vi "Runrate2.vi"() -> ()   [LabVIEW 2012]
uses:
  <vilib>/addons/database/Auxilliary.llb/DB Tools Cursor Type.ctl
  <vilib>/Utility/NIReport.llb/NI_report.lvclass
  <vilib>/addons/database/Connection.llb/DB Tools Open Connec (Path).vi
  <vilib>/addons/database/Connection.llb/Conn Execute.vi
  <vilib>/addons/database/Recordset.llb/Rec Fetch Recordset Data (R).vi
  <vilib>/addons/database/Recordset.llb/Rec Destroy - Connection.vi
  <vilib>/Utility/NIReport.llb/Append Text Table to Report (wrap).vi
  <vilib>/addons/database/_DB Variant To Data/Database Variant To Data.xnode
  <vilib>/addons/database/NI_Database_API.lvlib
  <vilib>/Utility/NIReport.llb/Excel/NI_Excel.lvclass
  <vilib>/addons/_office/NI_ReportGenerationToolkit.lvlib
panel:
  out "error out 2":errorcluster
  in  "Table Control":string[][](table)
  out "error out":errorcluster
  out "recordset data":variant[][](array[variant])
  out "array":string[][](array[string])
  out "transposed array":string[][](array[string])
  out "concatenated string":string
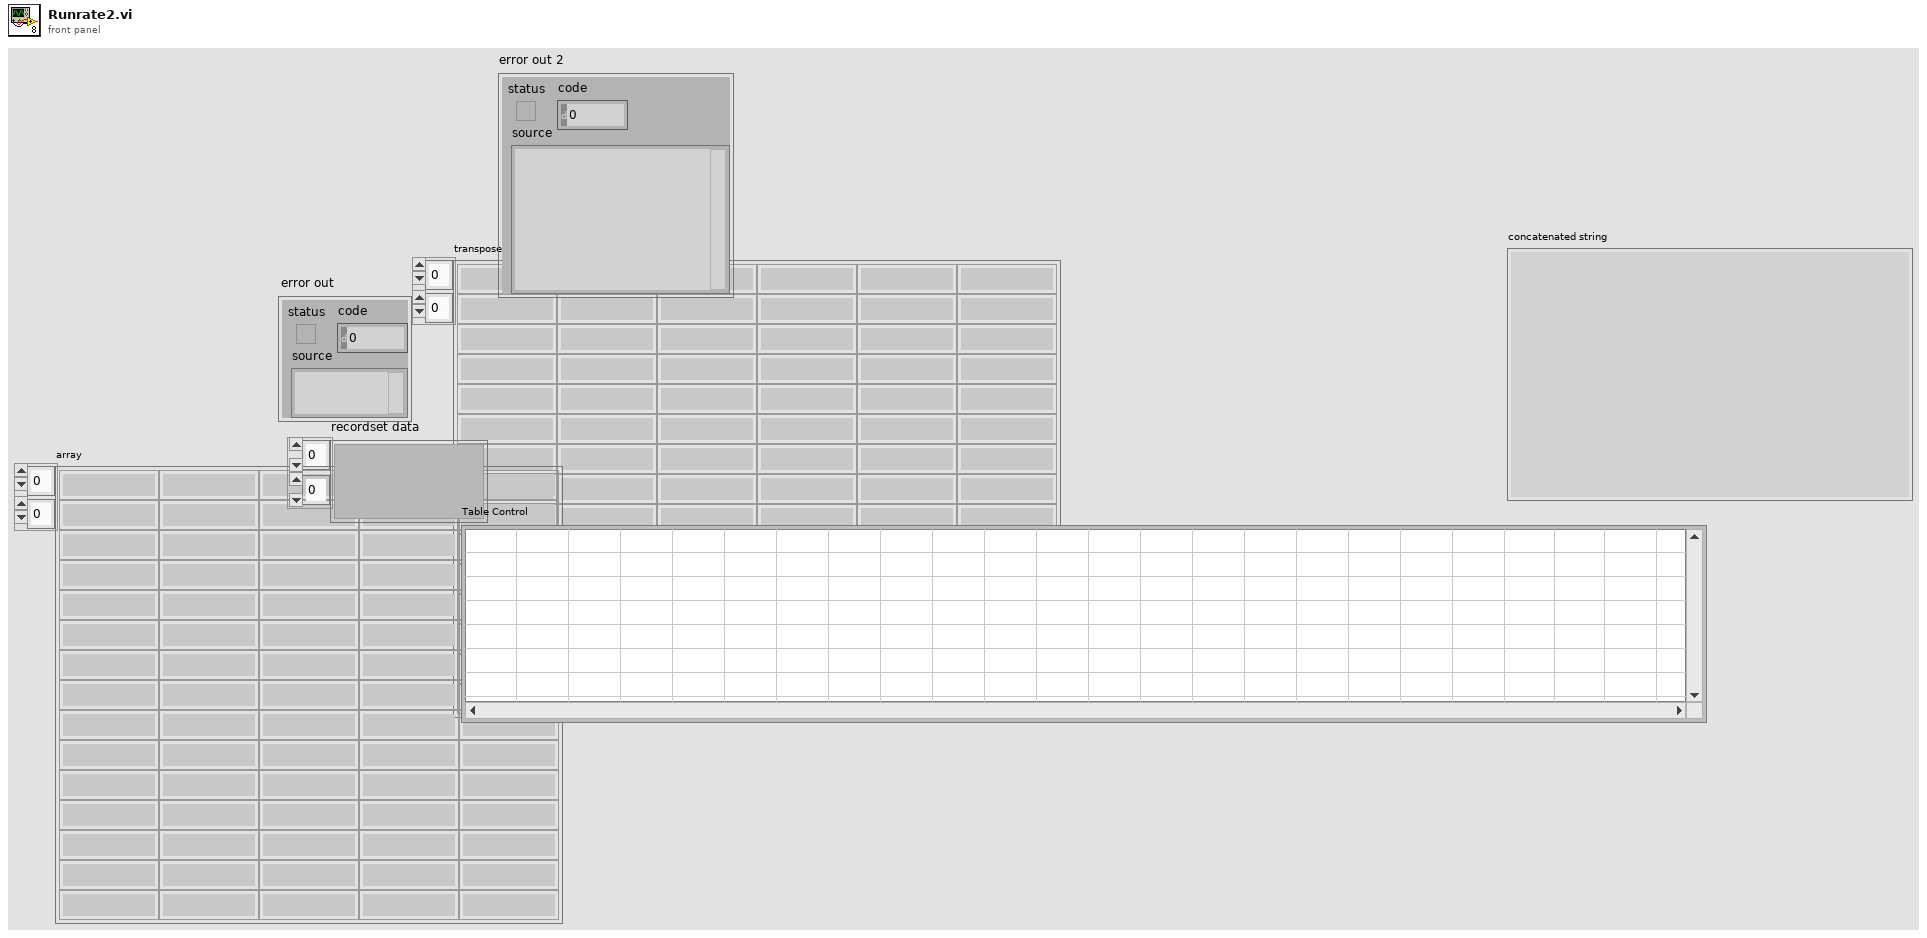
[diagram p1: front panel]
types:
  T1 = typedef "NI_Database_API.lvlib/DB Tools Cursor Type.ctl" = enum16{"forward-only", "keyset", "dynamic", "static"}
  T2 = typedef "NI_Database_API.lvlib/Conn ObjectReference.ctl" = refnum<k1>
  T3 = typedef "NI_Database_API.lvlib/Rec ObjectReference.ctl" = refnum<k1>
  T4 = enum16{"Standard Report", "HTML", "Word", "Excel"}
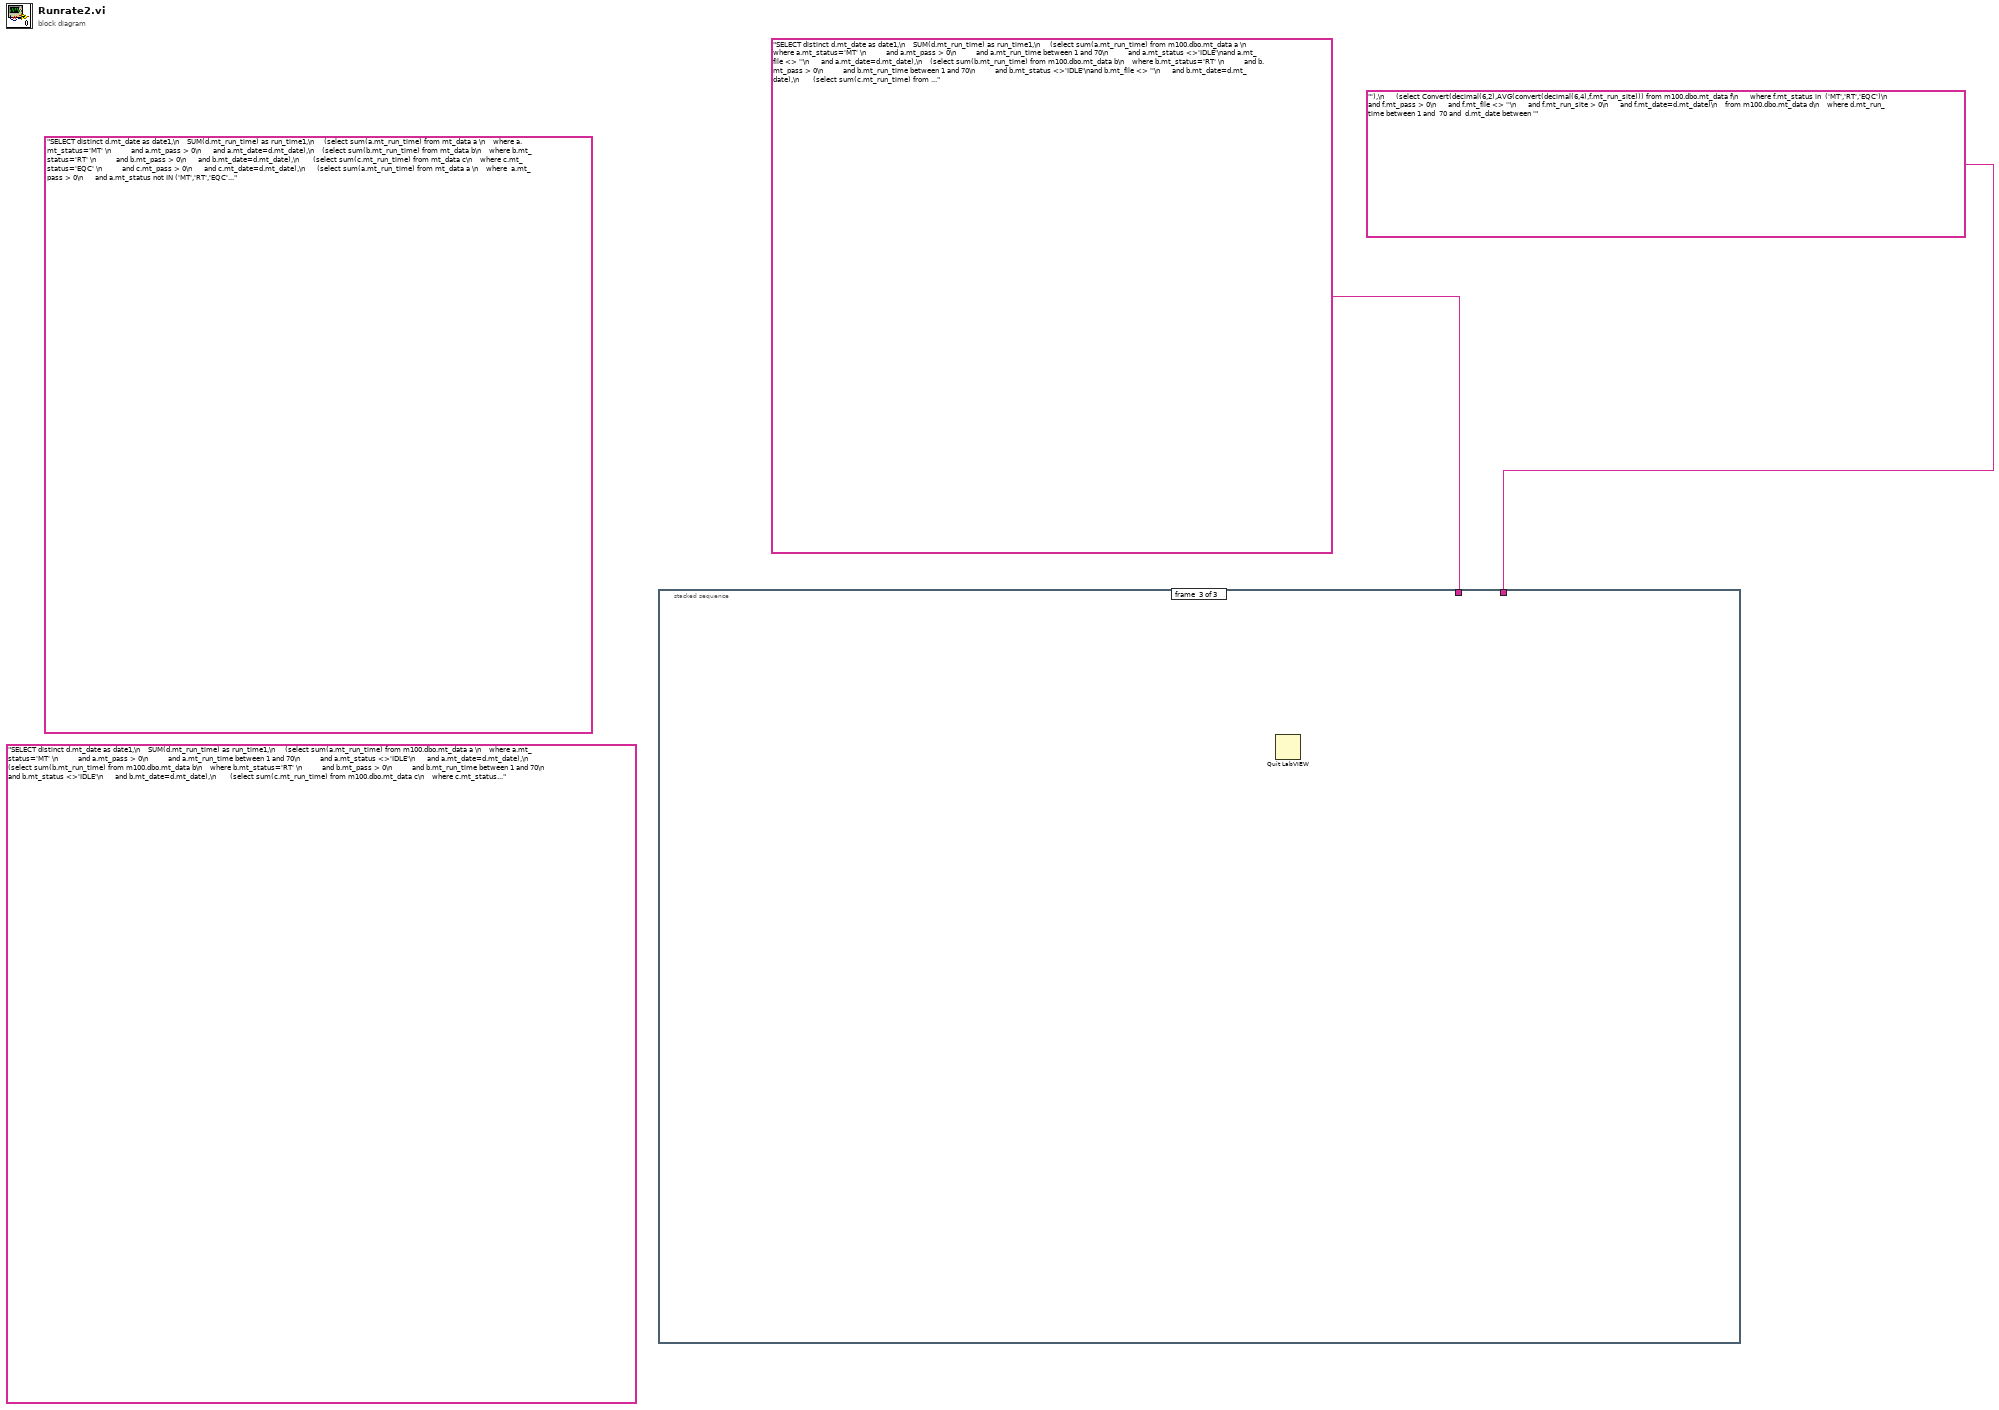
[diagram p0: block diagram]
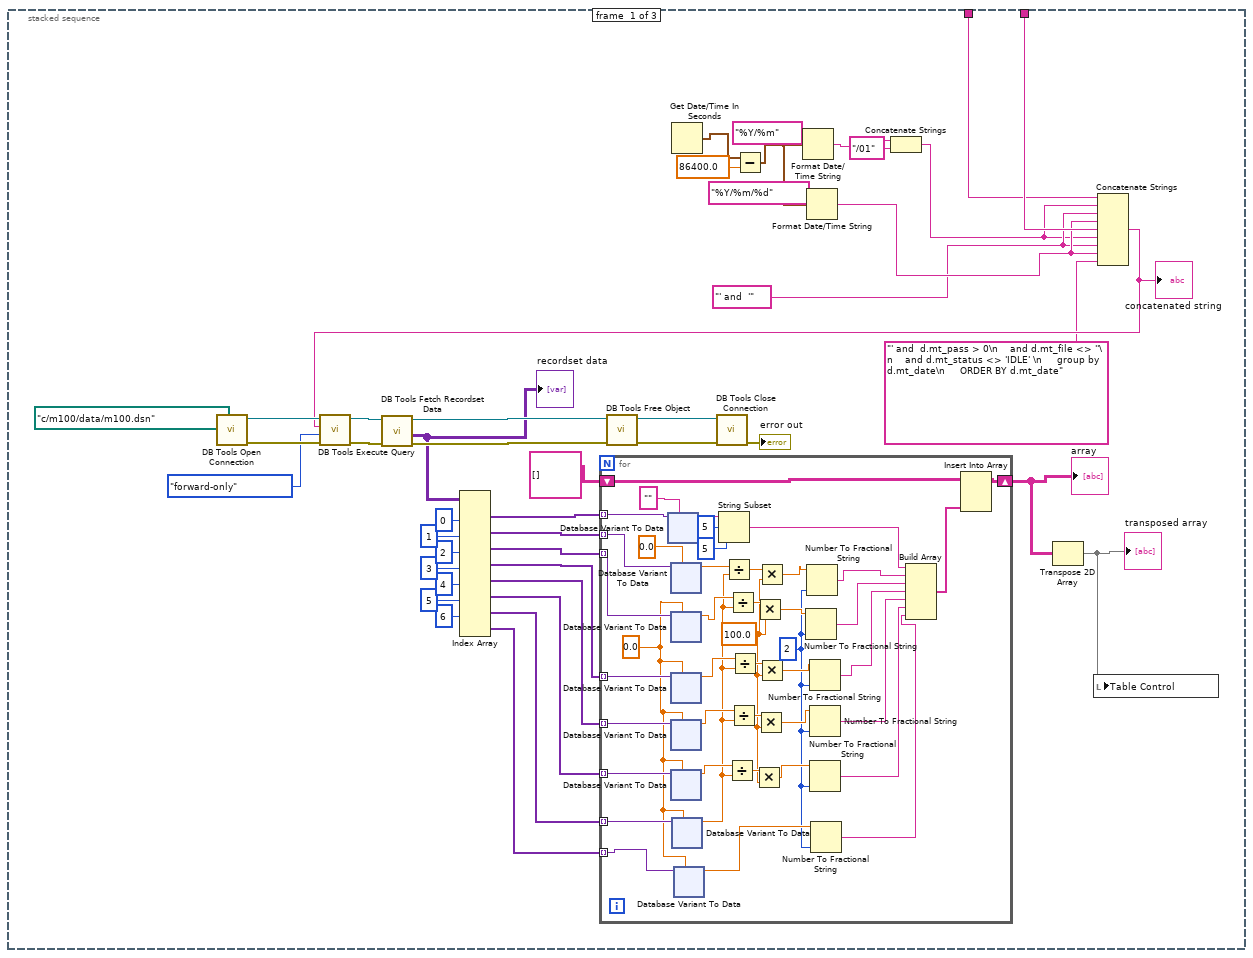
[diagram p2: hidden frame]
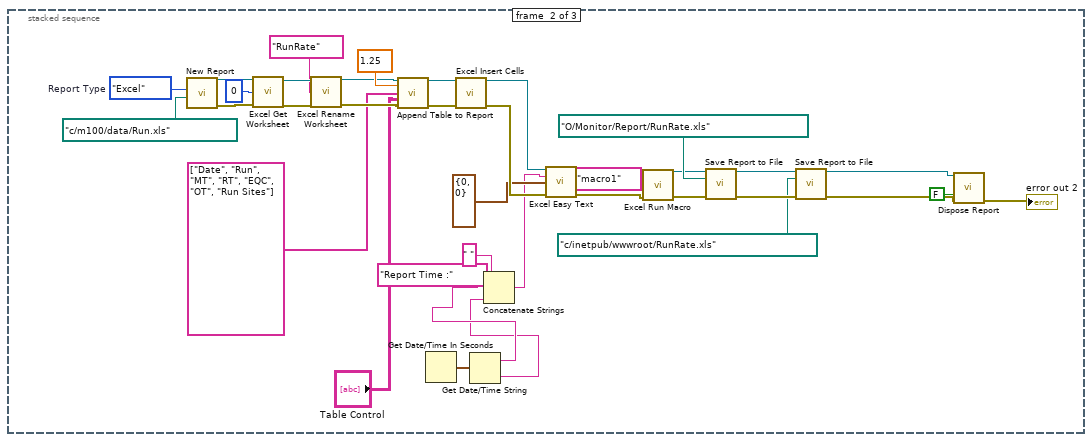
[diagram p3: hidden frame]
diagram:
  (unwired) "SELECT distinct d.mt_date as date1,\n    SUM(d.mt_run_time) as run_time1,\n     (select sum(a.mt_run_time) from mt_data a \n    where a.mt_status='MT' \n          and a.mt_pass > 0\n      and a.mt_date=d.mt_date),\n    (select sum(b.mt_run_time) from mt_data b\n    where b.mt_status='RT' \n          and b.mt_pass > 0\n      and b.mt_date=d.mt_date),\n       (select sum(c.mt_run_time) from mt_data c\n    where c.mt_status='EQC' \n          and c.mt_pass > 0\n      and c.mt_date=d.mt_date),\n      (select sum(a.mt_run_time) from mt_data a \n    where  a.mt_pass > 0\n      and a.mt_status not IN ('MT','RT','EQC')\n      and a.mt_run_time < 70\n      and a.mt_status <> 'IDLE'\n      and a.mt_file <> ''\n      and a.mt_date=d.mt_date),\n      (select COUNT(DISTINCT e.mt_machine)*1440 from mt_data e\n      where e.mt_date=d.mt_date),\n      (select Convert(decimal(6,2),AVG(convert(decimal(6,4),f.mt_run_site))) from mt_data f\n      where f.mt_status in  ('MT','RT','EQC')\n          and f.mt_pass > 0\n      and f.mt_file <> ''\n      and f.mt_run_site > 0\n      and f.mt_date=d.mt_date)\n    from mt_data d\n    where d.mt_run_time < 70 and  d.mt_date between '" ("SQL query")
  (unwired) "SELECT distinct d.mt_date as date1,\n    SUM(d.mt_run_time) as run_time1,\n     (select sum(a.mt_run_time) from m100.dbo.mt_data a \n    where a.mt_status='MT' \n          and a.mt_pass > 0\n          and a.mt_run_time between 1 and 70\n          and a.mt_status <>'IDLE'\n      and a.mt_date=d.mt_date),\n    (select sum(b.mt_run_time) from m100.dbo.mt_data b\n    where b.mt_status='RT' \n          and b.mt_pass > 0\n          and b.mt_run_time between 1 and 70\n          and b.mt_status <>'IDLE'\n      and b.mt_date=d.mt_date),\n       (select sum(c.mt_run_time) from m100.dbo.mt_data c\n    where c.mt_status='EQC' \n              and c.mt_run_time between 1 and 70\n          and c.mt_status <>'IDLE'\n          and c.mt_pass > 0\n      and c.mt_date=d.mt_date),\n      (select sum(a.mt_run_time) from m100.dbo.mt_data a \n    where  a.mt_pass > 0\n      and a.mt_status not IN ('MT','RT','EQC')\n                and a.mt_run_time between 1 and 70\n          and a.mt_status <>'IDLE'\n      and a.mt_file <> ''\n      and a.mt_date=d.mt_date),\n      (select COUNT(DISTINCT e.mt_machine)*1440 from m100.dbo.mt_data e\n      where e.mt_date between '2015/11/01' and  '2015/11/25' ),\n      (select Convert(decimal(6,2),AVG(convert(decimal(6,4),f.mt_run_site))) from m100.dbo.mt_data f\n      where f.mt_status in  ('MT','RT','EQC')\n          and f.mt_pass > 0\n      and f.mt_file <> ''\n      and f.mt_run_site > 0\n      and f.mt_date=d.mt_date)\n    from m100.dbo.mt_data d\n    where d.mt_run_time < 70 and  d.mt_date between '2015/11/01' and  '2015/11/25' and  d.mt_pass > 0\n    and d.mt_file <> ''\n    and d.mt_status <> 'IDLE' \n     group by d.mt_date\n     ORDER BY d.mt_date"
  n1 = stacked-sequence {
    tunnel: "SELECT distinct d.mt_date as date1,\n    SUM(d.mt_run_time) as run_time1,\n     (select sum(a.mt_run_time) from m100.dbo.mt_data a \n    where a.mt_status='MT' \n          and a.mt_pass > 0\n          and a.mt_run_time between 1 and 70\n          and a.mt_status <>'IDLE'\nand a.mt_file <> ''\n      and a.mt_date=d.mt_date),\n    (select sum(b.mt_run_time) from m100.dbo.mt_data b\n    where b.mt_status='RT' \n          and b.mt_pass > 0\n          and b.mt_run_time between 1 and 70\n          and b.mt_status <>'IDLE'\nand b.mt_file <> ''\n      and b.mt_date=d.mt_date),\n       (select sum(c.mt_run_time) from m100.dbo.mt_data c\n    where c.mt_status='EQC' \n              and c.mt_run_time between 1 and 70\n          and c.mt_status <>'IDLE'\nand c.mt_file <> ''\n          and c.mt_pass > 0\n      and c.mt_date=d.mt_date),\n      (select sum(a.mt_run_time) from m100.dbo.mt_data a \n    where  a.mt_pass > 0\n      and a.mt_status not IN ('MT','RT','EQC')\n                and a.mt_run_time between 1 and 70\n          and a.mt_status <>'IDLE'\n      and a.mt_file <> ''\n      and a.mt_date=d.mt_date),\n      (select COUNT(DISTINCT e.mt_machine)*1440 from m100.dbo.mt_data e\n      where e.mt_date between '" -> [w3 _ _]
    tunnel: "'),\n      (select Convert(decimal(6,2),AVG(convert(decimal(6,4),f.mt_run_site))) from m100.dbo.mt_data f\n      where f.mt_status in  ('MT','RT','EQC')\n          and f.mt_pass > 0\n      and f.mt_file <> ''\n      and f.mt_run_site > 0\n      and f.mt_date=d.mt_date)\n    from m100.dbo.mt_data d\n    where d.mt_run_time between 1 and  70 and  d.mt_date between '" -> [w7 _ _]
    frame #0 {
      w5 = "' and  '" ("string")
      n2 = call-poly <vilib>:"DB Tools Open Connection.vi"("connection information"=path "c:/m100/data/m100.dsn") -> ("error out"=w42:errorcluster, "connection reference"=w46:T2)  [unwired: 7 in]
      n3 = Get Date/Time In Seconds() -> (seconds since 1Jan1904=w13:timestamp)
      n4 = Subtract(x=w13, y=86400.0) -> (x-y=w8:timestamp)
      n5 = Format Date/Time String(time format string (%c)="%Y/%m", seconds (now)=w8) -> (date/time string=w11:string)  [unwired: 1 in]
      n6 = Format Date/Time String(time format string (%c)="%Y/%m/%d", seconds (now)=w8) -> (date/time string=w6:string)  [unwired: 1 in]
      n7 = Concatenate Strings(w11, "/01" ("string")) -> (w4:string)
      n8 = Concatenate Strings(w3, w4, w5, w6, w7, w4, w5, w6, "' and  d.mt_pass > 0\n    and d.mt_file <> ''\n    and d.mt_status <> 'IDLE' \n     group by d.mt_date\n     ORDER BY d.mt_date" ("string")) -> (w22:string)
      "concatenated string" <- w22
      n9 = call-poly <vilib>:"DB Tools Execute Query.vi"("error in (no error)"=w42, "cursor type"=DB_Tools_Cursor_Type."forward-only", "SQL query"=w22, "connection reference"=w46) -> ("error out"=w41:errorcluster, "recordset reference"=w45:T3)  [unwired: 4 in]
      n10 = call-poly <vilib>:"DB Tools Fetch Recordset Data.vi"("error in (no error)"=w41, "recordset reference"=w45) -> ("error out"=w40:errorcluster, "recordset data"=w35:variant[][], "recordset reference out"=w44:T3)  [unwired: 3 in]
      "recordset data" <- w35
      n11 = Index Array(array=w35, index (col) #1=0 ("disabled index (col)"), index (col) #2=1 ("index (col)"), index (col) #3=2 ("index (col)"), index (col) #4=3 ("index (col)"), index (col) #5=4 ("index (col)"), index (col) #6=5 ("index (col)"), index (col) #7=6 ("index (col)")) -> (element #1=w30:variant[], element #2=w29:variant[], element #3=w28:variant[], element #4=w26:variant[], element #5=w25:variant[], element #6=w20:variant[], element #7=w18:variant[], element #8=w15:variant[])  [unwired: 9 in]
      n12 = for {
        tunnel: w30 -> [w89] mode=indexing
        tunnel: w29 -> [w87] mode=indexing
        tunnel: w28 -> [w86] mode=indexing
        tunnel: w26 -> [w85] mode=indexing
        tunnel: w25 -> [w84] mode=indexing
        shift-right: [w78] -> w23
        shift-left: string[][] [] ("array") -> [w77]
        tunnel: w20 -> [w72] mode=indexing
        tunnel: w18 -> [w58] mode=indexing
        tunnel: w15 -> [w51] mode=indexing
        w55 = 100.0 ("y")
        w48 = i16 2 ("precision (6)")
        w50 = 0.0
        n13 = xnode "Database Variant To Data"("database variant"=w89, "type"="") -> ("data"=w76:string)  [unwired: 1 in, 1 out]
        n14 = xnode "Database Variant To Data"("database variant"=w87, "type"=0.0) -> ("data"=w54:dbl)  [unwired: 1 in, 1 out]
        n15 = xnode "Database Variant To Data"("database variant"=w86, "type"=w50) -> ("data"=w70:dbl)  [unwired: 1 in, 1 out]
        n16 = xnode "Database Variant To Data"("database variant"=w85, "type"=w50) -> ("data"=w66:dbl)  [unwired: 1 in, 1 out]
        n17 = xnode "Database Variant To Data"("database variant"=w84, "type"=w50) -> ("data"=w62:dbl)  [unwired: 1 in, 1 out]
        n18 = xnode "Database Variant To Data"("database variant"=w72, "type"=w50) -> ("data"=w59:dbl)  [unwired: 1 in, 1 out]
        n19 = xnode "Database Variant To Data"("database variant"=w58, "type"=w50) -> ("data"=w53:dbl)  [unwired: 1 in, 1 out]
        n20 = xnode "Database Variant To Data"("database variant"=w51, "type"=w50) -> ("data"=w49:dbl)  [unwired: 1 in, 1 out]
        n21 = String Subset(string=w76, offset (0)=5, length (rest)=5 ("length (rest)")) -> (substring=w75:string)
        n22 = Divide(x=w54, y=w53) -> (x/y=w57:dbl)
        n23 = Divide(x=w59, y=w53) -> (x/y=w61:dbl)
        n24 = Divide(x=w70, y=w53) -> (x/y=w69:dbl)
        n25 = Divide(x=w62, y=w53) -> (x/y=w65:dbl)
        n26 = Divide(x=w66, y=w53) -> (x/y=w67:dbl)
        n27 = Multiply(x=w61, y=w55) -> (x*y=w60:dbl)
        n28 = Multiply(x=w69, y=w55) -> (x*y=w68:dbl)
        n29 = Multiply(x=w65, y=w55) -> (x*y=w63:dbl)
        n30 = Multiply(x=w57, y=w55) -> (x*y=w56:dbl)
        n31 = Multiply(x=w67, y=w55) -> (x*y=w64:dbl)
        n32 = Number To Fractional String(number=w68, precision (6)=w48) -> (F-format string=w82:string)  [unwired: 2 in]
        n33 = Number To Fractional String(number=w56, precision (6)=w48) -> (F-format string=w52:string)  [unwired: 2 in]
        n34 = Number To Fractional String(number=w64, precision (6)=w48) -> (F-format string=w81:string)  [unwired: 2 in]
        n35 = Number To Fractional String(number=w63, precision (6)=w48) -> (F-format string=w80:string)  [unwired: 2 in]
        n36 = Number To Fractional String(number=w60, precision (6)=w48) -> (F-format string=w71:string)  [unwired: 2 in]
        n37 = Number To Fractional String(number=w49, precision (6)=w48) -> (F-format string=w47:string)  [unwired: 2 in]
        n38 = Build Array(w75, w52, w82, w81, w80, w71, w47) -> (w79:string[])
        n39 = Insert Into Array(array=w77, new element=w79) -> (w78:string[][])  [unwired: 2 in]
      }
      "array" <- w23
      n40 = call-poly <vilib>:"DB Tools Free Object.vi"("error in (no error)"=w40, "recordset reference"=w44) -> ("error out"=w39:errorcluster, "connection reference"=w43:T2)  [unwired: 8 in]
      n41 = call <vilib>:"DB Tools Close Connection.vi"("error in (no error)"=w39, "connection reference"=w43) -> ("error out"=→"error out":errorcluster)  [unwired: 5 in]
      n42 = Transpose 2D Array(2D array=w23) -> (transposed array=w16:string[][])
      "transposed array" <- w16
      n43 = local write "Table Control"(w16) -> ()
    }
    frame #1 {
      w382 = T4."Excel"  # Report Type
      n44 = call <vilib>:"New Report.vi"("report type"=w382, "template (empty)"=path "c:/m100/data/Run.xls" ("Report Template")) -> ("report out"=w377:refnum<class "NI_report.lvclass">, "error out"=w376:errorcluster)  [unwired: 12 in]
      n45 = call <vilib>:"Excel Get Worksheet.vi"("report in"=w377, "worksheet index (0)"=0, "error in (no error)"=w376) -> ("report out"=w374:refnum<class "NI_report.lvclass">, "error out"=w372:errorcluster)  [unwired: 11 in]
      n46 = call <vilib>:"Excel Rename Worksheet.vi"("report in"=w374, "worksheet name (\"\")"="RunRate" ("worksheet name (\"\")"), "error in (no error)"=w372) -> ("report out"=w373:refnum<class "NI_report.lvclass">, "error out"=w371:errorcluster)  [unwired: 11 in]
      n47 = call-poly <vilib>:"Append Table to Report.vi"("report in"=w373, "column width (1)"=1.25, "row headers"=string[] ["Date", "Run", "MT", "RT", "EQC", "OT", "Run Sites"], "text data"="Table Control", "error in (no error)"=w371) -> ("report out"=w379:refnum<class "NI_report.lvclass">, "error out"=w378:errorcluster)  [unwired: 7 in, 2 out]
      n48 = Get Date/Time In Seconds() -> (seconds since 1Jan1904=w365:timestamp)
      n49 = call <vilib>:"Excel Insert Cells.vi"("report in"=w379, "error in (no error)"=w378) -> ("report out"=w369:refnum<class "NI_report.lvclass">, "error out"=w368:errorcluster)  [unwired: 12 in]
      n50 = Get Date/Time String(seconds (now)=w365) -> (date string=w364:string, time string=w362:string)  [unwired: 2 in]
      n51 = Concatenate Strings("Report Time :" ("string"), w364, " " ("string"), w362) -> (w361:string)
      n52 = call <vilib>:"Excel Easy Text.vi"("report in"=w369, "text"=w361, "start (-1, -1)"=cluster{"row":i32, "column":i32} {"row"=0, "column"=0} ("end (-1, -1)"), "error in (no error)"=w368) -> ("report out"=w358:refnum<class "NI_report.lvclass">, "error out"=w357:errorcluster)  [unwired: 7 in, 3 out]
      n53 = call <vilib>:"Excel Run Macro.vi"("report in"=w358, "macro name"="macro1", "error in (no error)"=w357) -> ("report out"=w354:refnum<class "NI_report.lvclass">, "error out"=w353:errorcluster)  [unwired: 10 in, 1 out]
      n54 = call-dynamic "Save Report to File.vi"("report in"=w354, "report file path"=path "O:/Monitor/Report/RunRate.xls", "error in (no error)"=w353) -> ("report out"=w352:refnum<class "NI_report.lvclass">, "error out"=w351:errorcluster)  [unwired: 11 in]
      n55 = call-dynamic "Save Report to File.vi"("report in"=w352, "report file path"=path "c:/inetpub/wwwroot/RunRate.xls", "error in (no error)"=w351) -> ("report out"=w347:refnum<class "NI_report.lvclass">, "error out"=w346:errorcluster)  [unwired: 11 in]
      n56 = call-dynamic "Dispose Report.vi"("report in"=w347, "save changes? (F)"=FALSE, "error in (no error)"=w346) -> ("error out"=→"error out 2":errorcluster)  [unwired: 12 in]
    }
    frame #2 {
      n57 = Quit LabVIEW() -> ()  [unwired: 1 in]
    }
  }
